vi "Climber_Test.vi"(1 "Joystick_Out":T1) -> ()   [LabVIEW 2020]
uses:
  Utility VIs/Joystick_Controls.ctl
  Subsystems/Climber/Climber_Cluster.ctl
  Subsystems/Climber/Climber_Control_States.ctl
  Globals/Climber_Globals.vi
panel:
  in  "Inner Pivot Left Trigger Deadzone Size":dbl=0.05 format="%#_13g"
  in  "Inner Pivot Right Trigger Deadzone Size":dbl=0.05 format="%#_13g"
  in  "Outer Elevator Deadzone Size":dbl=0.05 format="%#_13g"
  in  "Outer Pivot Deadzone Size":dbl=0.05 format="%#_13g"
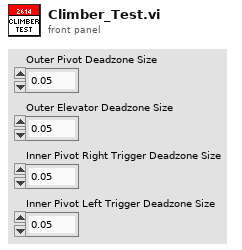
[diagram p1: front panel]
types:
  T1 = typedef "Joystick_Controls.ctl" = cluster{"Pilot Left Joystick X":dbl, "Pilot Left Joystick Y":dbl, "Pilot A Button":bool, "Pilot B Button":bool, "Pilot X Button":bool, "Pilot Y Button":bool, "Pilot Left Bumper":bool, "Pilot Right Bumper":bool, "Pilot View Button":bool, "Pilot Menu Button":bool, "Pilot Left Joystick Press":bool, "Pilot Right Joystick Press":bool, "Pilot Left Trigger":dbl, "Pilot Right Joystick X":dbl, "Pilot Right Joystick Y":dbl, "Pilot Right Trigger":dbl, "Copilot Left Joystick X":dbl, "Copilot Left Joystick Y":dbl, "Copilot A Button":bool, "Copilot B Button":bool, "Copilot X Button":bool, "Copilot Y Button":bool, "Copilot Left Bumper":bool, "Copilot Right Bumper":bool, "Copilot View Button":bool, "Copilot Menu Button":bool, "Copilot Left Joystick Press":bool, "Copilot Right Joystick Press":bool, "Copilot Left Trigger":dbl, "Copilot Right Joystick X":dbl, "Copilot Right Joystick Y":dbl, "Copilot Right Trigger":dbl, "Pilot D-pad North":bool, "Pilot D-pad South":bool, "Pilot D-pad East":bool, "Pilot D-pad West":bool, "Pilot D-pad NE ":bool, "Pilot D-pad SE":bool, "Pilot D-pad SW":bool, "Pilot D-pad NW":bool, "CoPilot D-pad North":bool, "CoPilot D-pad South":bool, "CoPilot D-pad East":bool, "CoPilot D-pad West":bool, "CoPilot D-pad NE":bool, "CoPilot D-pad SE":bool, "CoPilot D-pad SW":bool, "CoPilot D-pad NW":bool, "Pilot Left Trigger Pressed":bool, "Pilot Right Trigger Pressed":bool, "CoPilot Left Trigger Pressed":bool, "CoPilot Right Trigger Pressed":bool}
  T2 = typedef "Climber_Cluster.ctl" = cluster{"Control_State":T3, "Outer_Arm_Pivot_Throttle":dbl, "Outer_Arm_Elevator_Throttle":dbl, "Inner_Arm_Pivot_Throttle":dbl, "Enable_Climber_Sequence":bool}
  T3 = typedef "Climber_Control_States.ctl" = enum16{"No-Op", "Manual_%Vbus", "Climbing_Sequence"}
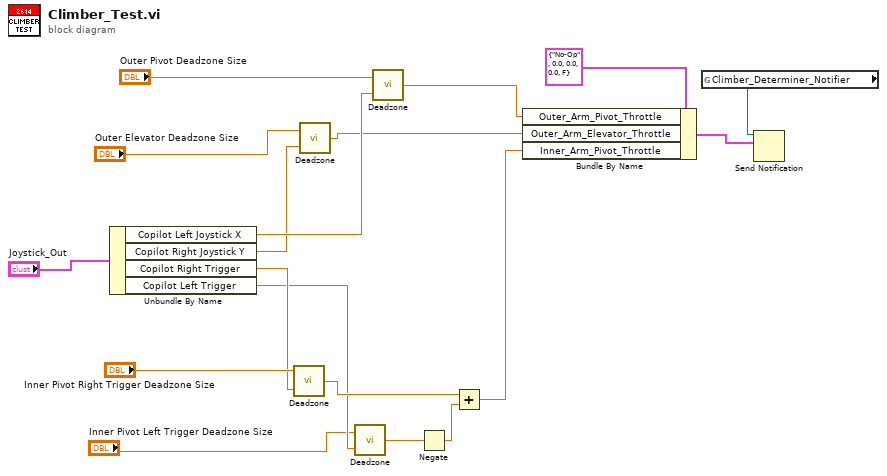
[diagram p0: block diagram]
diagram:
  n1 = Unbundle By Name("Joystick_Out") -> ("Copilot Left Joystick X"=w11:dbl, "Copilot Right Joystick Y"=w9:dbl, "Copilot Right Trigger"=w6:dbl, "Copilot Left Trigger"=w4:dbl)
  n2 = call "Deadzone.vi"("Joystick Value Input"=w6, "Deadzone Size"="Inner Pivot Right Trigger Deadzone Size") -> ("Corrected Joystick Value"=w5:dbl)  [unwired: 1 in]
  n3 = call "Deadzone.vi"("Joystick Value Input"=w9, "Deadzone Size"="Outer Elevator Deadzone Size") -> ("Corrected Joystick Value"=w1:dbl)  [unwired: 1 in]
  n4 = call "Deadzone.vi"("Joystick Value Input"=w4, "Deadzone Size"="Inner Pivot Left Trigger Deadzone Size") -> ("Corrected Joystick Value"=w2:dbl)  [unwired: 1 in]
  n5 = call "Deadzone.vi"("Joystick Value Input"=w11, "Deadzone Size"="Outer Pivot Deadzone Size") -> ("Corrected Joystick Value"=w10:dbl)  [unwired: 1 in]
  n6 = Negate(x=w2) -> (-x=w13:dbl)
  n7 = Add(x=w5, y=w13) -> (x+y=w16:dbl)
  n8 = Bundle By Name(cluster=T2 {"Control_State"=enum."No-Op", "Outer_Arm_Pivot_Throttle"=0.0, "Outer_Arm_Elevator_Throttle"=0.0, "Inner_Arm_Pivot_Throttle"=0.0, "Enable_Climber_Sequence"=FALSE} ("Climber_Cluster"), "Outer_Arm_Pivot_Throttle"=w10, "Outer_Arm_Elevator_Throttle"=w1, "Inner_Arm_Pivot_Throttle"=w16) -> (w17:T2)
  n9 = global read "Climber_Globals.vi" "Climber_Determiner_Notifier"() -> (w18:refnum<notifier>)
  n10 = Send Notification(notification=w17, notifier=w18) -> ()  [unwired: 1 in, 2 out]
